vi "sub_ReadConfiguration.vi"(6 "create file if necessary? (T)":bool=TRUE caption="必要时创建文件？(T)", 7 "Section Formatted Cluster Type":variant, 8 "error in (no error)":errorcluster, 11 "configuration file path":path caption="配置文件的路径") -> (0 "error out":errorcluster caption="错误输出", 3 "数据":variant)   [LabVIEW 2013, in "0_SystemCOnfiguration.lvlib"]
uses:
  0_SystemCOnfiguration.lvlib
  <vilib>/Utility/config.llb/NI_LVConfig.lvlib
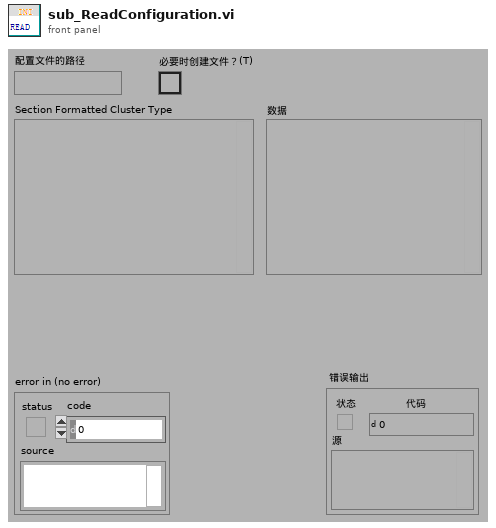
[diagram p1: front panel]
types:
  T1 = typedef "NI_LVConfig.lvlib/Config Data RefNum.ctl" = refnum<k1>
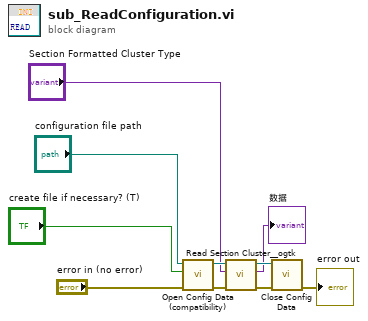
[diagram p0: block diagram]
diagram:
  n1 = call <vilib>:"Open Config Data (compatibility).vi"("error in (no error)"="error in (no error)", "create file if necessary (T)"="create file if necessary? (T)", "configuration file path"="configuration file path") -> ("error out"=w10:errorcluster, "refnum"=w9:T1)  [unwired: 6 in, 1 out]
  n2 = call <userlib>:"Read Section Cluster__ogtk.vi"("error in (no error)"=w10, "Section Formatted Cluster Type"="Section Formatted Cluster Type", "refnum"=w9) -> ("error out"=w7:errorcluster, "Section Formatted Cluster"=→"数据":variant, "dup refnum"=w8:T1)  [unwired: 4 in, 2 out]
  n3 = call <vilib>:"Close Config Data.vi"("error in (no error)"=w7, "refnum"=w8) -> ("error out"=→"error out":errorcluster)  [unwired: 8 in, 1 out]
